vi "Child Path.vi"(10 "Name":string, 11 "Remote Directory":string) -> (3 "String":string)   [LabVIEW 2017, in "FTP.lvlib" / "FTP.lvclass"]
uses:
  FTP.lvclass
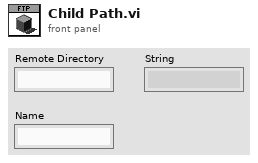
[diagram p1: front panel]
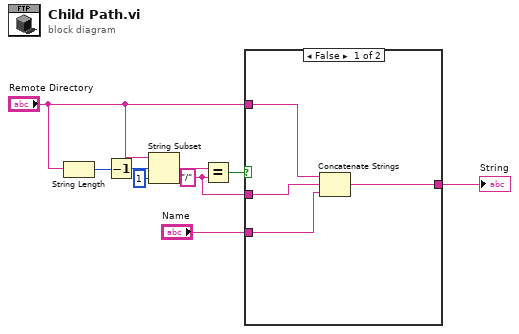
[diagram p0: block diagram]
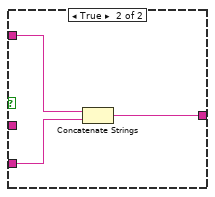
[diagram p2: hidden frame]
diagram:
  w1 = "/" ("y")
  n1 = String Length(string="Remote Directory") -> (length=w6:i32)
  n2 = Decrement(x=w6) -> (x-1=w5:i32)
  n3 = String Subset(string="Remote Directory", offset (0)=w5, length (rest)=1 ("length (rest)")) -> (substring=w3:string)
  n4 = Equal?(x=w3, y=w1) -> (x = y?=w2:bool)
  n5 = case shown="False" w2 {
    tunnel: [w10 w16] -> w9
    tunnel: "Name" -> [w11 w15]
    tunnel: "Remote Directory" -> [w13 w14]
    tunnel: w1 -> [w12 _]
    frame False {
      n6 = Concatenate Strings(w13, w12, w11) -> (w10:string)
    }
    frame True {
      n7 = Concatenate Strings(w14, w15) -> (w16:string)
    }
  }
  "String" <- w9
